vi "test Multiple Clients - Secure.vi"(8 "error in (no error)":errorcluster, 11 "TestCase in":refnum<class "test Multiple Clients.lvclass">) -> (0 "error out":errorcluster, 3 "TestCase out":refnum<class "test Multiple Clients.lvclass">)   [LabVIEW 2013, in "test Multiple Clients.lvclass"]
uses:
  test Multiple Clients.lvclass
  dotNET SSL Socket/dotNET SSL Socket/PFX Certificate.ctl
  dotNET SSL Socket/dotNET SSL Listener/dotNET Listener.lvclass
  dotNET SSL Socket/dotNET SSL Client/dotNET SSL Client Socket.lvclass
  dotNET SSL Socket/dotNET SSL Server/dotNET SSL Server.lvclass/dotNET SSL Server.ctl
  dotNET SSL Socket/dotNET SSL Server/dotNET SSL Server.lvclass
  dotNET SSL Socket/dotNET SSL Server/Write Server Certificate.vi
  <vilib>/addons/_JKI Toolkits/VI Tester/TestCase.llb/TestCase.lvclass
  dotNET SSL Socket/dotNET TCP Socket/dotNET TCP Socket.lvclass
  dotNET SSL Socket/dotNET SSL Socket/dotNET SSL Socket.lvclass
panel:
  out "Sent":string[](array[string])
  out "Received by Server":string[](array[string])
  out "Returned":string[](array[string])
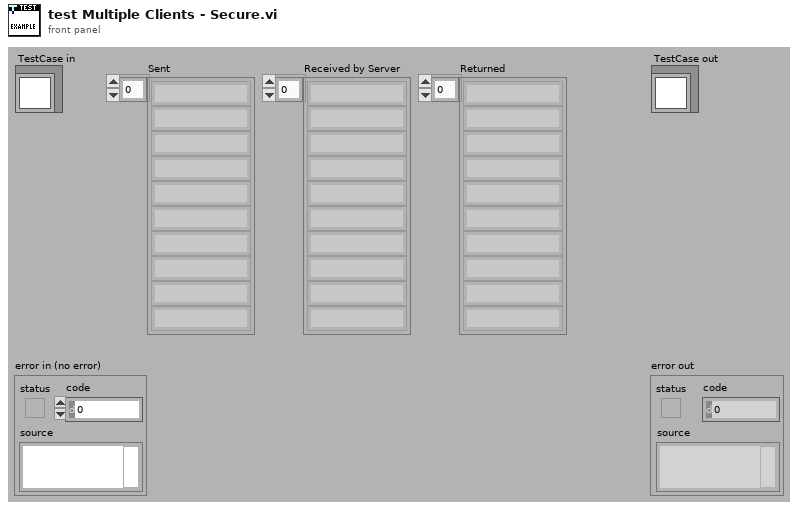
[diagram p1: front panel]
types:
  T1 = typedef "dotNET SSL Socket.lvlib/dotNET SSL Socket.lvclass/PFX Certificate.ctl" = cluster{"PFX Certificate":path, "PFX Password":string}
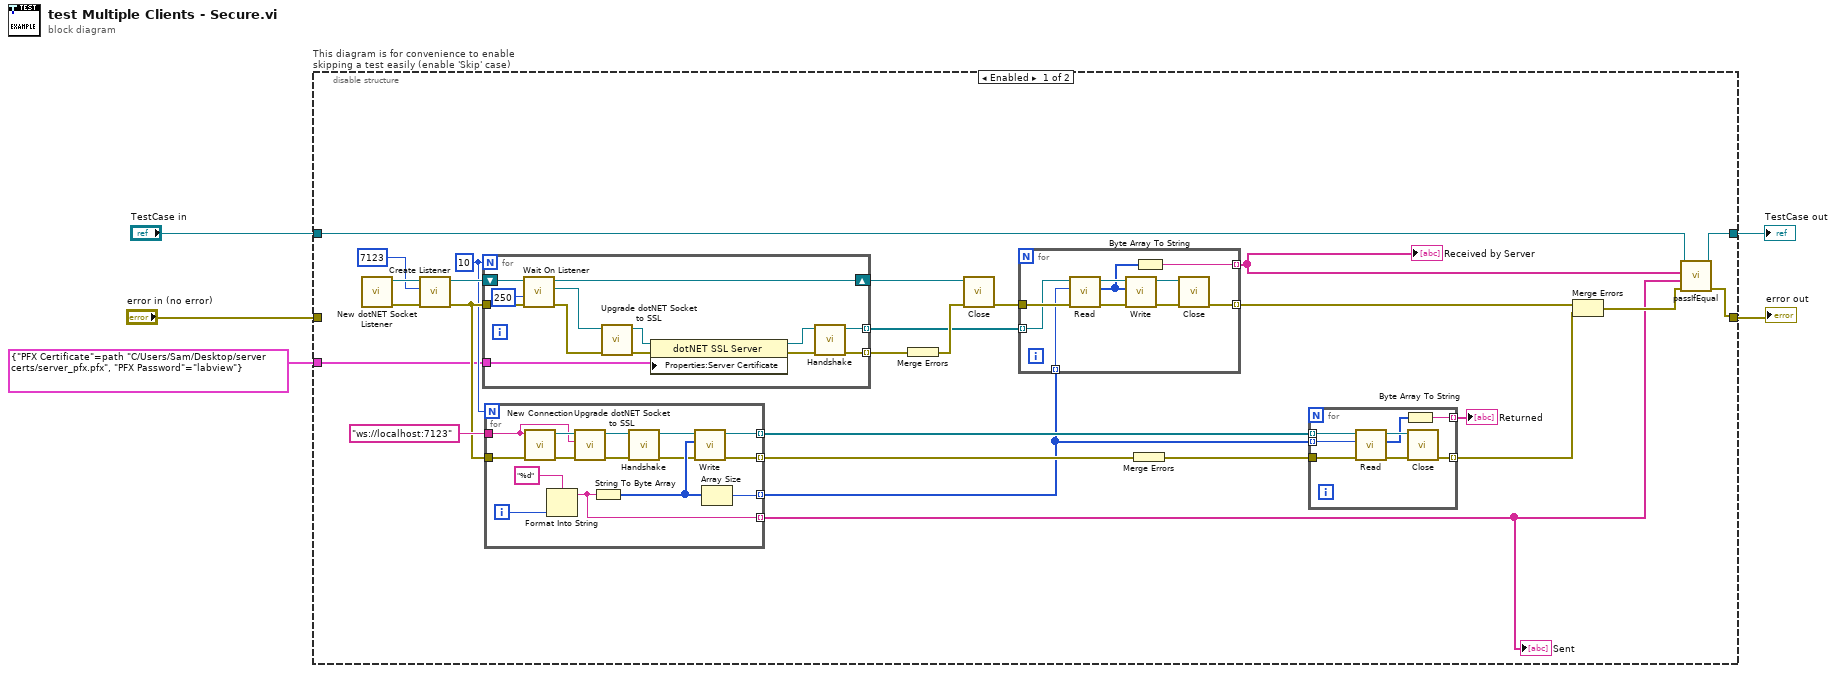
[diagram p0: block diagram]
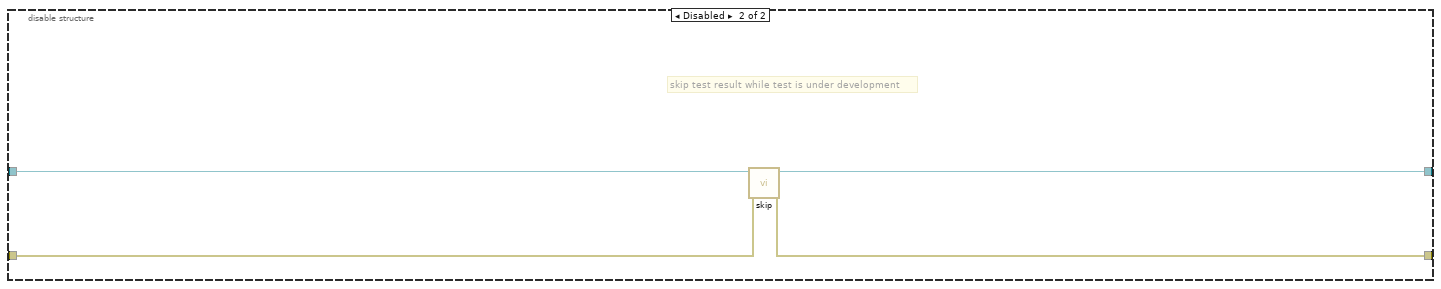
[diagram p2: hidden frame]
diagram:
  n1 = disable-structure "This diagram is for convenience to enable skipping a test easily (enable 'Skip' case)" shown="Enabled" {
    disable-tunnel: "TestCase in" -> [w31 w81]
    disable-tunnel: [w30 w79] -> w2
    disable-tunnel: [w29 w80] -> w4
    disable-tunnel: "error in (no error)" -> [_ w78]
    disable-tunnel: T1 {"PFX Certificate"=path "C:/Users/Sam/Desktop/server certs/server_pfx.pfx", "PFX Password"="labview"} ("Server Certificate") -> [w6 _]
    frame Enabled {
      w16 = 10
      n2 = call "New dotNET Socket Listener.vi"() -> ("error out"=w28:errorcluster, "dotNET Listener out"=w27:refnum<class "dotNET Listener.lvclass">)  [unwired: 10 in]
      n3 = call-dynamic "Create Listener.vi"("error in (no error)"=w28, "Port"=u16 7123, "dotNET Listener in"=w27) -> ("error out"=w23:errorcluster, "dotNET Listener out"=w26:refnum<class "dotNET Listener.lvclass">)  [unwired: 7 in]
      n4 = for {
        N: w16 -> [_]
        tunnel: w23 -> [w76]
        shift-right: [w75] -> w21
        shift-left: w26 -> [w77]
        tunnel: [w67] -> w22 mode=indexing
        tunnel: [w66] -> w19 mode=indexing
        tunnel: w6 -> [w65]
        n5 = call-dynamic "Wait On Listener.vi"("error in (no error)"=w76, "timeout ms (5000)"=250, "dotNET Listener in"=w77) -> ("error out"=w72:errorcluster, "Socket out"=w73:refnum<class "Socket.lvclass">, "dotNET Listener out"=w75:refnum<class "dotNET Listener.lvclass">)  [unwired: 6 in]
        n6 = call "Upgrade dotNET Socket to SSL.vi"("error in (no error)"=w72, "Socket in"=w73) -> ("error out"=w70:errorcluster, "dotNET SSL Socket out"=w71:refnum<class "dotNET SSL Server.lvclass">)  [unwired: 8 in]
        n7 = property class="dotNET SSL Server"(reference=w71, error in=w70, "Properties:Server Certificate"=w65) -> (reference out=w69:refnum<class "dotNET SSL Server.lvclass">, error out=w68:errorcluster)
        n8 = call-dynamic "Handshake.vi"("error in (no error)"=w68, "dotNET SSL Socket in"=w69) -> ("error out"=w67:errorcluster, "dotNET SSL Socket out"=w66:refnum<class "dotNET SSL Server.lvclass">)  [unwired: 8 in]
      }
      n9 = for {
        N: w16 -> [_]
        tunnel: "ws://localhost:7123" ("Hostname / URL") -> [w54]
        tunnel: w23 -> [w64]
        tunnel: [w60] -> w9 mode=indexing
        tunnel: [w59] -> w7 mode=indexing
        tunnel: [w58] -> w14 mode=indexing
        tunnel: [w57] -> w13 mode=indexing
        i -> [w63]
        n10 = call "New Connection.vi"("error in (no error)"=w64, "Hostname / URL"=w54) -> ("error out"=w55:errorcluster, "dotNET TCP Socket out"=w56:refnum<class "dotNET TCP Socket.lvclass">)  [unwired: 8 in]
        n11 = Format Into String(format string="%d", w63) -> (resulting string=w59:string)  [unwired: 2 in, 1 out]
        n12 = call "Upgrade dotNET Socket to SSL.vi"("error in (no error)"=w55, "Hostname / URL"=w54, "dotNET TCP Socket in"=w56) -> ("error out"=w53:errorcluster, "dotNET SSL Client Socket out"=w52:refnum<class "dotNET SSL Client Socket.lvclass">)  [unwired: 7 in]
        n13 = String To Byte Array(string=w59) -> (unsigned byte array=w61:u8[])
        n14 = call-dynamic "Handshake.vi"("error in (no error)"=w53, "dotNET SSL Client Socket in"=w52) -> ("error out"=w51:errorcluster, "dotNET SSL Client Socket out"=w50:refnum<class "dotNET SSL Client Socket.lvclass">)  [unwired: 8 in]
        n15 = call-dynamic "Write.vi"("error in (no error)"=w51, "Bytes to write"=w61, "dotNET SSL Socket in"=w50) -> ("error out"=w57:errorcluster, "dotNET SSL Socket out"=w58:refnum<class "dotNET SSL Client Socket.lvclass">)  [unwired: 6 in, 1 out]
        n16 = Array Size(array=w61) -> (size(s)=w60:i32)
      }
      "Sent" <- w7
      n17 = Merge Errors(w22) -> (w20:errorcluster)
      n18 = call-dynamic "Close.vi"("error in (no error)"=w20, "dotNET Listener in"=w21) -> ("error out"=w18:errorcluster)  [unwired: 9 in]
      n19 = for {
        tunnel: w19 -> [w48] mode=indexing
        tunnel: w18 -> [w49]
        tunnel: w9 -> [w47] mode=indexing
        tunnel: [w46] -> w17 mode=indexing
        tunnel: [w40] -> w15 mode=indexing
        n20 = call-dynamic "Read.vi"("error in (no error)"=w49, "# bytes to read"=w47, "dotNET SSL Socket in"=w48) -> ("error out"=w44:errorcluster, "Read Bytes"=w41:u8[], "dotNET SSL Socket out"=w45:refnum<class "dotNET SSL Server.lvclass">)  [unwired: 6 in]
        n21 = call-dynamic "Write.vi"("error in (no error)"=w44, "Bytes to write"=w41, "dotNET SSL Socket in"=w45) -> ("error out"=w43:errorcluster, "dotNET SSL Socket out"=w42:refnum<class "dotNET SSL Server.lvclass">)  [unwired: 6 in, 1 out]
        n22 = Byte Array To String(unsigned byte array=w41) -> (string=w46:string)
        n23 = call-dynamic "Close.vi"("error in (no error)"=w43, "dotNET SSL Socket in"=w42) -> ("error out"=w40:errorcluster)  [unwired: 9 in]
      }
      "Received by Server" <- w17
      n24 = Merge Errors(w13) -> (w12:errorcluster)
      n25 = for {
        tunnel: w14 -> [w39] mode=indexing
        tunnel: w12 -> [w38]
        tunnel: [w35] -> w11 mode=indexing
        tunnel: w9 -> [w34] mode=indexing
        tunnel: [w32] -> w8 mode=indexing
        n26 = call-dynamic "Read.vi"("error in (no error)"=w38, "# bytes to read"=w34, "dotNET SSL Socket in"=w39) -> ("error out"=w37:errorcluster, "Read Bytes"=w33:u8[], "dotNET SSL Socket out"=w36:refnum<class "dotNET SSL Client Socket.lvclass">)  [unwired: 6 in]
        n27 = Byte Array To String(unsigned byte array=w33) -> (string=w32:string)
        n28 = call-dynamic "Close.vi"("error in (no error)"=w37, "dotNET SSL Socket in"=w36) -> ("error out"=w35:errorcluster)  [unwired: 9 in]
      }
      "Returned" <- w8
      n29 = Merge Errors(w15, w11) -> (w10:errorcluster)
      n30 = call-dynamic "passIfEqual.vi"("error in (no error)"=w10, "y"=w7, "x"=w17, "TestCase in"=w31) -> ("error out"=w29:errorcluster, "TestCase out"=w30:refnum<class "test Multiple Clients.lvclass">)  [unwired: 6 in]
    }
    frame Disabled {
      # "skip test result while test is under development"
      n31 = call <vilib>:"skip.vi"("error in (no error)"=w78, "TestCase in"=w81) -> ("error out"=w80:errorcluster, "TestCase out"=w79:refnum<class "test Multiple Clients.lvclass">)  [unwired: 8 in]
    }
  }
  "error out" <- w4
  "TestCase out" <- w2
